vi "Constrained Non-Linear Fit (Best of All).vi"(0 "Y Array":dbl[](array[numeric]), 1 "f(x,a)":refnum<vi>, 2 "Data":variant, 3 "Fitting Method":T2=enum."Best of All", 4 "Optimal Offset Selection Criterion":T1, 5 "X Array":dbl[](array[numeric]), 7 "Weights":dbl[](array[numeric]), 9 "Guess Fitted Parameters":dbl[](array[numeric]), 11 "error in (no error)":errorcluster, 12 "Termination Criteria":T4={"Max Iterations"=1000, "Max Function Calls"=10000, "Max Time"=1000.0, "Function Tolerance"=1e-06, "Parameter Tolerance"=1e-06, "Gradient Tolerance"=1e-06, "Min Lambda"=1e-06, "Max Lambda"=1e-06, "Initial Tick Count"=0}, 13 "Fitted parameter bounds":T7, 14 "Fitting Algorithm":T3) -> (6 "Fit Output":T8={"best nonlinear fit"=[], "best fit parameters"=[], "R^2"=0.0, "RMSE"=0.0, "error out"={"status"=FALSE, "code"=0, "source"=""}, "Fitting Method"=enum."Least Square", "number of function calls"=0, "number of iterations"=0, "covariance"=[], "Chi 2"=0.0, "DOF"=0, "Fit Convergence Criterion"=enum."Continue", "Fitting Algorithm"=enum."Levenberg-Marquardt", "Weighted Fit"=enum."Unweighted", "Gradient"=0.0, "|Delta Chi 2|"=0.0, "|Delta Chi 2|/Chi 2"=0.0, "Max |Delta a| /|a|"=0.0, "Lambda"=-1.0, "RSS"=0.0, "AIC"=0.0, "BIC"=0.0, "Max number of function calls"=0, "Max number of iterations"=0, "IRF"={"X Array"=[], "Y Array"=[]}, "IRF Normalization Factor"=0.0, "Decay Normalization Factor"=0.0, "Number of offset fits"=0, "Weighted Chi2"=-1.0, "Unweighted Chi2"=-1.0}, 8 "Fit Results (Stats)":T6[](array[typedef]), 10 "Fit Aborted?":bool, 15 "Error Out":errorcluster)   [LabVIEW 2021, in "Fits.lvlib"]
uses:
  Fits.lvlib
  Non-linear Fit Output v4.ctl
  Nonlinear Fit Method.ctl
  <vilib>/Analysis/Matrix/Datatypes/RealMatrix.ctl
  Convergence Criteria.ctl
  Non-linear Fitting Algorithm.ctl
  IRF(X)PSED/Fit Weights Type v2.ctl
  Graphs/XY Graph/XY Graph Plot Data.ctl
  My Fit Stopping Criteria.ctl
  Non-linear Fitting Method v2.ctl
  Fit Results (statistics).ctl
  Optimal Offset Selection Criterion.ctl
  Decay Convolution/Fit Control Data.ctl
  Decay Convolution/Fit Control Data v2.ctl
  IRF(X)PSED/Decay Fit Parameters In List.ctl
  Decay Convolution/Decay Model.ctl
  Abort Fit Global.vi
  <userlib>/_OpenG.lib/array/array.llb/Remove Duplicates from 1D Array (DBL)__ogtk.vi
  <vilib>/Analysis/NI_AALPro.lvlib
  <vilib>/Analysis/Matrix/NI_Matrix.lvlib
  Graphs/XY Graph/XY Graph Add-Ons.lvlib
  Error/Error.lvlib
  <userlib>/_OpenG.lib/array/array.llb/openg_array.lvlib
panel:
  in  "Cluster":T5={"Optimal Offset Selection Criterion"=enum."Min Chi^2", "Fitting Method"=enum."Best of All", "Fitting Algorithm"=enum."Levenberg-Marquardt", "Termination Criteria"={"Max Iterations"=1000, "Max Function Calls"=10000, "Max Time"=1000.0, "Function Tolerance"=1e-06, "Parameter Tolerance"=1e-06, "Gradient Tolerance"=1e-06, "Min Lambda"=1e-06, "Max Lambda"=1e-06, "Initial Tick Count"=0}, "Fitted parameter bounds"={"parameter minimum"=[], "parameter maximum"=[]}}
  # "see the AlliGator License on the block diagram (Ctrl+E or Window:Show Block Diagram)"
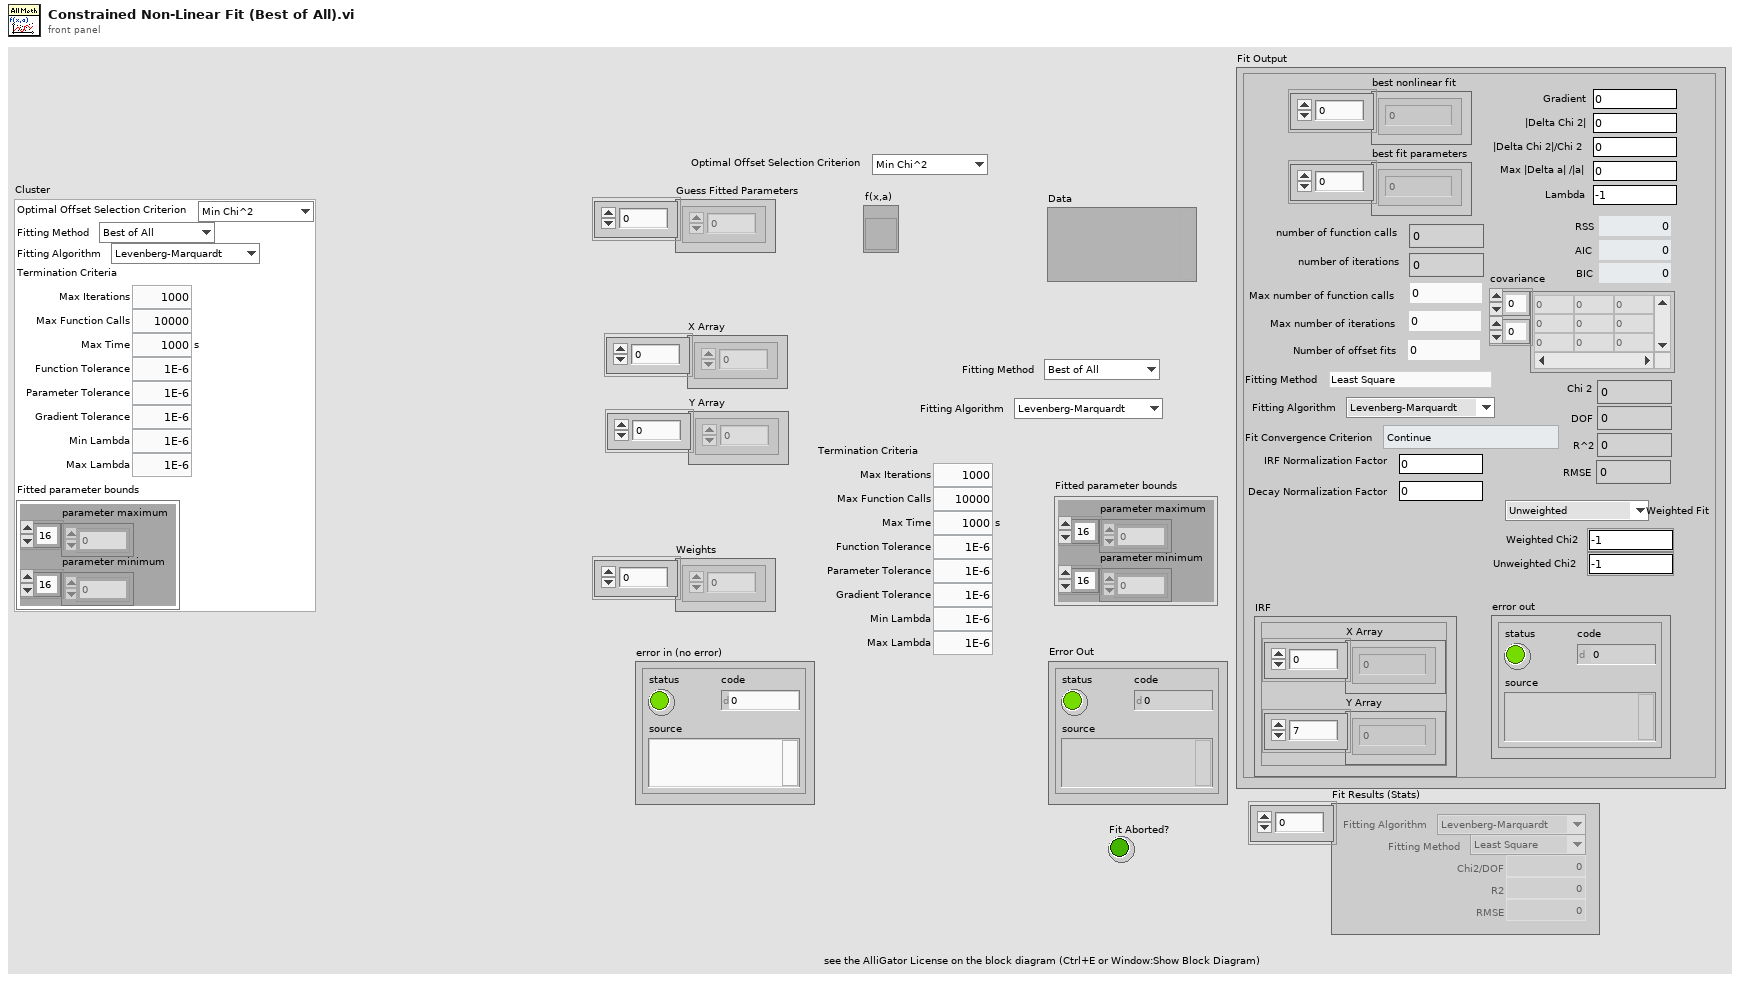
[diagram p1: front panel]
types:
  T1 = typedef "Fits.lvlib/Optimal Offset Selection Criterion.ctl" = enum16{"Min Chi^2", "Max R^2"}
  T2 = typedef "Fits.lvlib/Non-linear Fitting Method v2.ctl" = enum16{"Least Square", "Least Absolute Residual", "Bisquare", "MLE", "-", "Best of All"}
  T3 = typedef "Fits.lvlib/Non-linear Fitting Algorithm.ctl" = enum16{"Levenberg-Marquardt", "Trust-Region Dogleg"}
  T4 = typedef "Fits.lvlib/My Fit Stopping Criteria.ctl" = cluster{"Max Iterations":i32, "Max Function Calls":i32, "Max Time":dbl[unit], "Function Tolerance":dbl, "Parameter Tolerance":dbl, "Gradient Tolerance":dbl, "Min Lambda":dbl, "Max Lambda":dbl, "Initial Tick Count":u32}
  T5 = cluster{"Optimal Offset Selection Criterion":T1, "Fitting Method":T2, "Fitting Algorithm":T3, "Termination Criteria":T4, "Fitted parameter bounds":cluster{"parameter minimum":dbl[], "parameter maximum":dbl[]}}
  T6 = typedef "Fits.lvlib/Fit Results (statistics).ctl" = cluster{"Chi2/DOF":dbl, "R2":dbl, "RMSE":dbl, "Fitting Method":T2, "Fitting Algorithm":T3}
  T7 = cluster{"parameter minimum":dbl[], "parameter maximum":dbl[]}
  T8 = typedef "Fits.lvlib/Non-linear Fit Output v4.ctl" = cluster{"best nonlinear fit":dbl[], "best fit parameters":dbl[], "R^2":dbl, "RMSE":dbl, "error out":errorcluster, "Fitting Method":T9, "number of function calls":i32, "number of iterations":i32, "covariance":T10, "Chi 2":dbl, "DOF":i32, "Fit Convergence Criterion":T11, "Fitting Algorithm":T3, "Weighted Fit":T12, "Gradient":dbl, "|Delta Chi 2|":dbl, "|Delta Chi 2|/Chi 2":dbl, "Max |Delta a| /|a|":dbl, "Lambda":dbl, "RSS":dbl, "AIC":dbl, "BIC":dbl, "Max number of function calls":i32, "Max number of iterations":i32, "IRF":T13, "IRF Normalization Factor":dbl, "Decay Normalization Factor":dbl, "Number of offset fits":i32, "Weighted Chi2":dbl, "Unweighted Chi2":dbl}
  T9 = typedef "Fits.lvlib/Nonlinear Fit Method.ctl" = enum16{"Least Square", "Least Absolute Residual", "Bisquare", "MLE"}
  T10 = typedef "NI_Matrix.lvlib/RealMatrix.ctl" = dbl[][]
  T11 = typedef "Fits.lvlib/Convergence Criteria.ctl" = enum16{"Continue", "Tolerances Exceeded", "Max Time Exceeded", "Max Iterations Exceeded", "Max Function Evaluations Exceeded", "Scale Range Exceeded"}
  T12 = typedef "Fits.lvlib/Fit Weights Type v2.ctl" = enum16{"Unweighted", "1/Variance (Neyman)", "1/Variance (Pearson)", "Best of All"}
  T13 = typedef "XY Graph Add-Ons.lvlib/XY Graph Plot Data.ctl" = cluster{"X Array":dbl[], "Y Array":dbl[]}
  T14 = typedef "Fits.lvlib/Fit Control Data v2.ctl" = cluster{"IRF":T13, "Laser Period":dbl, "SYNC Period":dbl, "Fixed Parameter Names":T15[], "Fixed Parameter Values":dbl[], "Fitted Parameter Names":T15[], "Fit Model":T16}
  T15 = typedef "Fits.lvlib/Decay Fit Parameters In List.ctl" = enum16{"Offset", "Baseline", "A_1", "tau_1", "A_2", "tau_2"}
  T16 = typedef "Fits.lvlib/Decay Model.ctl" = enum16{"1-Exponential", "2-Exponentials"}
  T17 = typedef "Fits.lvlib/Fit Control Data.ctl" = cluster{"IRF":T13, "Laser Period":dbl, "SYNC Period":dbl}
  T18 = typedef "Fits.lvlib/Fit Statistics v3.ctl" = cluster{"# Iterations":i32, "# Function Calls":i32, "Chi2":dbl, "Chi2/DOF":dbl, "Fit Convergence Criterion":T11, "Gradient":dbl, "|Delta Chi 2|":dbl, "|Delta Chi 2|/Chi 2":dbl, "Max |Delta a| /|a|":dbl, "Lambda":dbl, "Weighted Chi2":dbl, "Unweighted Chi2":dbl}
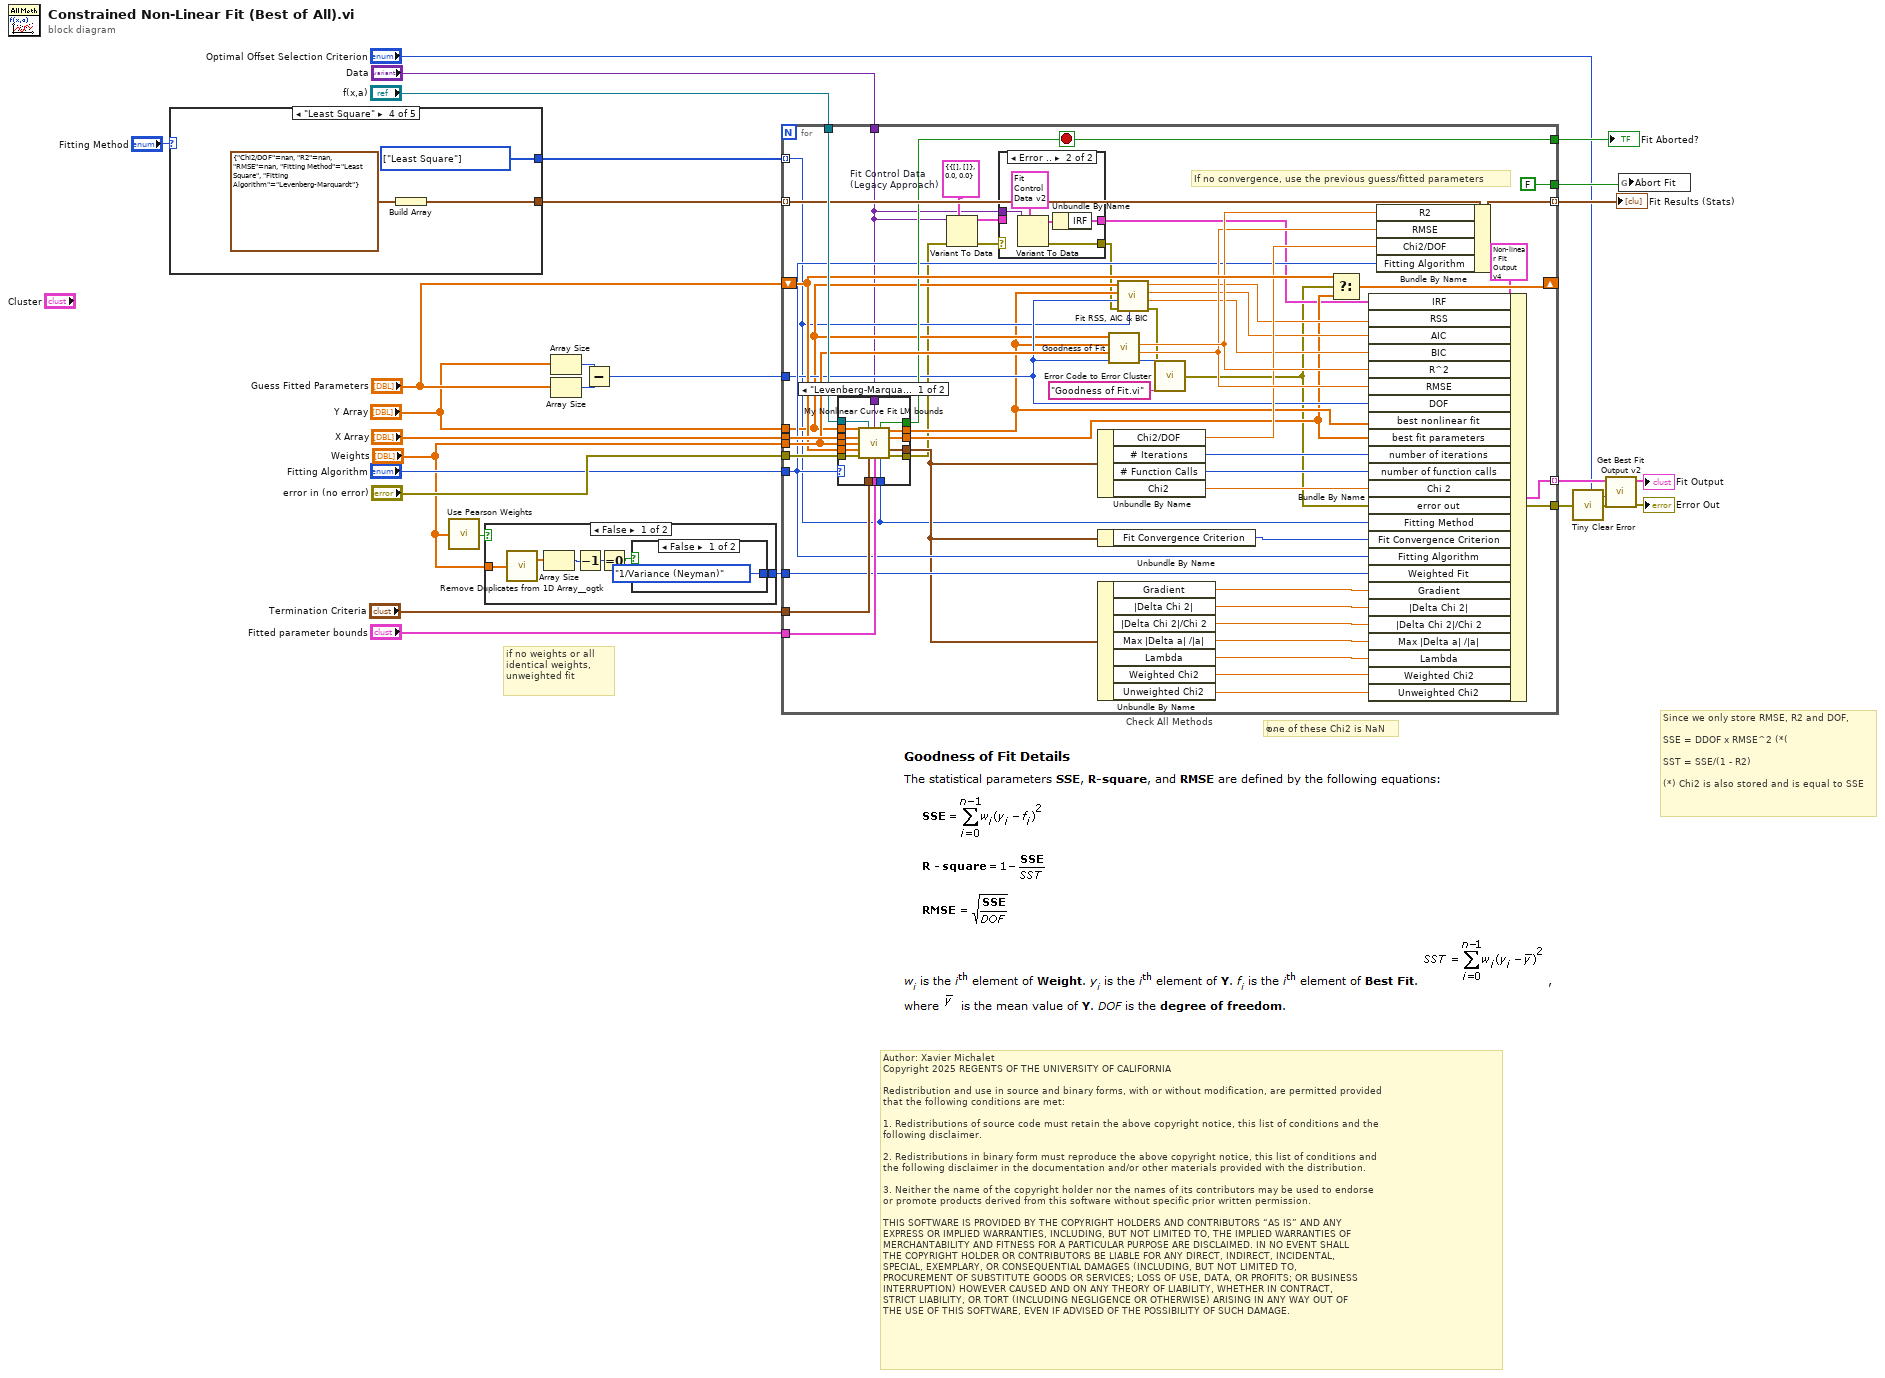
[diagram p0: block diagram]
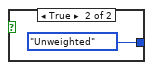
[diagram p2: hidden frame]
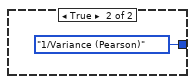
[diagram p3: hidden frame]
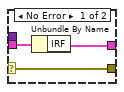
[diagram p4: hidden frame]
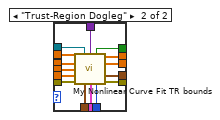
[diagram p5: hidden frame]
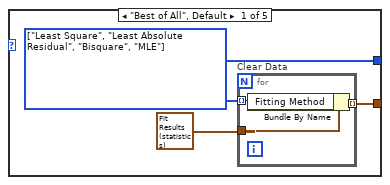
[diagram p6: hidden frame]
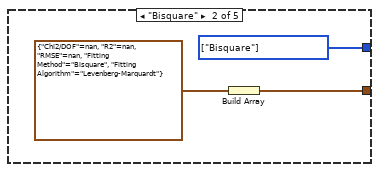
[diagram p7: hidden frame]
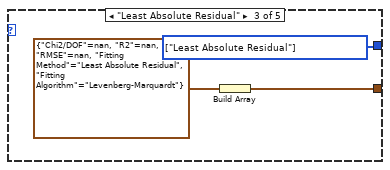
[diagram p8: hidden frame]
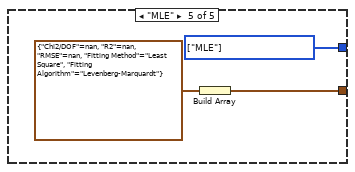
[diagram p9: hidden frame]
diagram:
  # "one of these Chi2 is NaN"
  # "one of these Chi2 is NaN"
  # "Author: Xavier Michalet\nCopyright 2025 REGENTS OF THE UNIVERSITY OF CALIFORNIA\n\nRedistribution and use in source and binary forms, with or without modification, are permitted provided\nthat the following conditions are met:\n\n1. Redistributions of source code must retain the above copyright notice, this list of conditions and the\nfollowing disclaimer.\n\n2. Redistributions in binary form must reproduce the above copyright notice, this list of conditions and\nthe following disclaimer in the documentation and/or other materials provided with the distribution.\n\n3. Neither the name of the copyright holder nor the names of its contributors may be used to endorse \nor promote products derived from this software without specific prior written permission.\n\nTHIS SOFTWARE IS PROVIDED BY THE COPYRIGHT HOLDERS AND CONTRIBUTORS “AS IS” AND ANY \nEXPRESS OR IMPLIED WARRANTIES, INCLUDING, BUT NOT LIMITED TO, THE IMPLIED WARRANTIES OF\nMERCHANTABILITY AND FITNESS FOR A PARTICULAR PURPOSE ARE DISCLAIMED. IN NO EVENT SHALL\nTHE COPYRIGHT HOLDER OR CONTRIBUTORS BE LIABLE FOR ANY DIRECT, INDIRECT, INCIDENTAL, \nSPECIAL, EXEMPLARY, OR CONSEQUENTIAL DAMAGES (INCLUDING, BUT NOT LIMITED TO, \nPROCUREMENT OF SUBSTITUTE GOODS OR SERVICES; LOSS OF USE, DATA, OR PROFITS; OR BUSINESS\nINTERRUPTION) HOWEVER CAUSED AND ON ANY THEORY OF LIABILITY, WHETHER IN CONTRACT, \nSTRICT LIABILITY, OR TORT (INCLUDING NEGLIGENCE OR OTHERWISE) ARISING IN ANY WAY OUT OF\nTHE USE OF THIS SOFTWARE, EVEN IF ADVISED OF THE POSSIBILITY OF SUCH DAMAGE."
  # "if no weights or all identical weights, unweighted fit"
  # "Since we only store RMSE, R2 and DOF,\n\nSSE = DDOF x RMSE^2 (*(\n\nSST = SSE/(1 - R2)\n\n(*) Chi2 is also stored and is equal to SSE"
  n1 = case shown="\"Least Square\"" "Fitting Method" {
    tunnel: [w30 w36 w39 w42 w45] -> w11
    tunnel: [w29 w35 w38 w41 w44] -> w9
    frame "Best of All", Default {
      w30 = T9[] [enum."Least Square", enum."Least Absolute Residual", enum."Bisquare", enum."MLE"] items=["Least Square", "Least Absolute Residual", "Bisquare", "MLE"] ("Array")
      n2 = for "Clear Data" {
        tunnel: w30 -> [w32] mode=indexing
        tunnel: T6 {"Chi2/DOF"=nan, "R2"=nan, "RMSE"=nan, "Fitting Method"=enum."Least Square", "Fitting Algorithm"=enum."Levenberg-Marquardt"} ("Fit Statistics") -> [w33]
        tunnel: [w31] -> w29 mode=indexing
        n3 = Bundle By Name(cluster=w33, "Fitting Method"=w32) -> (w31:T6)
      }
    }
    frame "Bisquare" {
      w36 = T9[] [enum."Bisquare"] items=["Least Square", "Least Absolute Residual", "Bisquare", "MLE"] ("Array")
      n4 = Build Array(T6 {"Chi2/DOF"=nan, "R2"=nan, "RMSE"=nan, "Fitting Method"=enum."Bisquare", "Fitting Algorithm"=enum."Levenberg-Marquardt"} ("Fit Statistics")) -> (w35:T6[])
    }
    frame "Least Absolute Residual" {
      w39 = T9[] [enum."Least Absolute Residual"] items=["Least Square", "Least Absolute Residual", "Bisquare", "MLE"] ("Array")
      n5 = Build Array(T6 {"Chi2/DOF"=nan, "R2"=nan, "RMSE"=nan, "Fitting Method"=enum."Least Absolute Residual", "Fitting Algorithm"=enum."Levenberg-Marquardt"} ("Fit Statistics")) -> (w38:T6[])
    }
    frame "Least Square" {
      w42 = T9[] [enum."Least Square"] items=["Least Square", "Least Absolute Residual", "Bisquare", "MLE"] ("Array")
      n6 = Build Array(T6 {"Chi2/DOF"=nan, "R2"=nan, "RMSE"=nan, "Fitting Method"=enum."Least Square", "Fitting Algorithm"=enum."Levenberg-Marquardt"} ("Fit Statistics")) -> (w41:T6[])
    }
    frame "MLE" {
      w45 = T9[] [enum."MLE"] items=["Least Square", "Least Absolute Residual", "Bisquare", "MLE"] ("Array")
      n7 = Build Array(T6 {"Chi2/DOF"=nan, "R2"=nan, "RMSE"=nan, "Fitting Method"=enum."Least Square", "Fitting Algorithm"=enum."Levenberg-Marquardt"} ("Fit Statistics")) -> (w44:T6[])
    }
  }
  n8 = call "Use Pearson Weights.vi"("Weight"="Weights") -> ("Use Pearson Weight"=w1:bool)
  n9 = case shown="False" w1 {
    tunnel: [w47 Fit_Weights_Type_v2."1/Variance (Pearson)" ("Weighted Fit")] -> w3
    tunnel: "Weights" -> [w46 _]
    frame False {
      n10 = call-poly <userlib>:"Remove Duplicates from 1D Array__ogtk.vi"("Input Array"=w46) -> ("Output Array"=w51:dbl[])  [unwired: 1 out]
      n11 = Array Size(array=w51) -> (size(s)=w50:i32)
      n12 = Decrement(x=w50) -> (x-1=w49:i32)
      n13 = Equal To 0?(x=w49) -> (x = 0?=w48:bool)
      n14 = case shown="False" w48 {
        tunnel: [Fit_Weights_Type_v2."1/Variance (Neyman)" ("Weighted Fit") Fit_Weights_Type_v2."Unweighted" ("Weighted Fit")] -> w47
        frame False {
        }
        frame True {
        }
      }
    }
    frame True {
    }
  }
  n15 = Array Size(array="Y Array") -> (size(s)=w17:i32)
  n16 = Array Size(array="Guess Fitted Parameters") -> (size(s)=w18:i32)
  n17 = Subtract(x=w17, y=w18) -> (x-y=w24:i32)
  n18 = for "Check All Methods" {
    tunnel: "Y Array" -> [w74]
    tunnel: "X Array" -> [w104]
    tunnel: "Weights" -> [w101]
    shift-right: [w98] -> _
    shift-left: "Guess Fitted Parameters" -> [w99]
    tunnel: "f(x,a)" -> [w102]
    tunnel: "Data" -> [w58]
    tunnel: w11 -> [w70] mode=indexing
    tunnel: w24 -> [w75]
    tunnel: [w100] -> w26 mode=indexing
    tunnel: "error in (no error)" -> [w103]
    tunnel: "Termination Criteria" -> [w89]
    tunnel: "Fitted parameter bounds" -> [w97]
    tunnel: [w84] -> w13
    tunnel: [FALSE ("Abort Fit")] -> w10
    tunnel: w9 -> [w88] mode=indexing
    tunnel: [w87] -> w8 mode=indexing
    tunnel: "Fitting Algorithm" -> [w83]
    tunnel: w3 -> [w82]
    tunnel: [w63] -> w6
    stop <- w84 stop-if-true
    w61 = T17 {"IRF"={"X Array"=[], "Y Array"=[]}, "Laser Period"=0.0, "SYNC Period"=0.0}  # Fit Control Data (Legacy Approach)
    # "If no convergence, use the previous guess/fitted parameters"
    n19 = case shown="\"Levenberg-Marquardt\", Default" w83 {
      tunnel: w104 -> [w127 w142]
      tunnel: w103 -> [w126 w141]
      tunnel: w102 -> [w125 w140]
      tunnel: w58 -> [w124 w139]
      tunnel: w74 -> [w123 w138]
      tunnel: w101 -> [w122 w137]
      tunnel: w99 -> [w121 w136]
      tunnel: w97 -> [w120 w135]
      tunnel: [w119 w134] -> w69
      tunnel: [w118 w133] -> w68
      tunnel: [w117 w132] -> w62
      tunnel: w70 -> [w116 w131]
      tunnel: w89 -> [w115 w130]
      tunnel: [w114 w129] -> w81
      tunnel: [w113 w128] -> w84
      frame "Levenberg-Marquardt", Default {
        n20 = call "My Nonlinear Curve Fit LM bounds.vi"("Y"=w123, "f(x,a)"=w125, "data"=w124, "X"=w127, "Weight"=w122, "initial parameters"=w121, "error in (no error)"=w126, "Termination Criteria"=w115, "parameter bounds"=w120, "NL Fit Method"=w116) -> ("Fit Aborted?"=w113:bool, "best nonlinear fit"=w119:dbl[], "best fit parameters"=w118:dbl[], "Fit Statistics"=w114:T18, "error out"=w117:errorcluster)  [unwired: 1 out]
      }
      frame "Trust-Region Dogleg" {
        n21 = call "My Nonlinear Curve Fit TR bounds.vi"("Y"=w138, "f(x,a)"=w140, "data"=w139, "X"=w142, "Weight"=w137, "initial parameters"=w136, "error in (no error)"=w141, "Termination Criteria"=w130, "parameter bounds"=w135, "method"=w131) -> ("Fit Aborted?"=w128:bool, "best nonlinear fit"=w134:dbl[], "best fit parameters"=w133:dbl[], "Fit Statistics"=w129:T18, "error out"=w132:errorcluster)  [unwired: 1 out]
      }
    }
    n22 = Variant To Data(error in=w62, type=w61, Variant=w58) -> (data=w59:T17, error out=w60:errorcluster)
    n23 = case shown="Error .." w60 {
      selector: w60 -> [w105 _]
      tunnel: [w106 w110] -> w67
      tunnel: [w105 w109] -> w66
      tunnel: w59 -> [w107 _]
      tunnel: w58 -> [_ w108]
      frame No Error {
        n24 = Unbundle By Name(w107) -> ("IRF"=w106:T13)
      }
      frame Error {
        n25 = Variant To Data(type=T14 {"IRF"={"X Array"=[], "Y Array"=[]}, "Laser Period"=0.0, "SYNC Period"=0.0, "Fixed Parameter Names"=[], "Fixed Parameter Values"=[], "Fitted Parameter Names"=[], "Fit Model"=enum."1-Exponential"} ("Fit Control Data"), Variant=w108) -> (data=w111:T14, error out=w109:errorcluster)  [unwired: 1 in]
        n26 = Unbundle By Name(w111) -> ("IRF"=w110:T13)
      }
    }
    n27 = Unbundle By Name(w81) -> ("Chi2/DOF"=w93:dbl, "# Iterations"=w92:i32, "# Function Calls"=w91:i32, "Chi2"=w86:dbl)
    n28 = Unbundle By Name(w81) -> ("Fit Convergence Criterion"=w85:T11)
    n29 = Unbundle By Name(w81) -> ("Gradient"=w80:dbl, "|Delta Chi 2|"=w79:dbl, "|Delta Chi 2|/Chi 2"=w78:dbl, "Max |Delta a| /|a|"=w77:dbl, "Lambda"=w76:dbl, "Weighted Chi2"=w56:dbl, "Unweighted Chi2"=w55:dbl)
    n30 = call <vilib>:"Goodness of Fit.vi"("degree of freedom"=w75, "Weight"=w101, "Best Fit"=w69, "Y"=w74) -> ("error"=w65:i32, "RMSE"=w94:dbl, "R-square"=w95:dbl)  [unwired: 4 in, 1 out]
    n31 = call "Fit RSS, AIC & BIC.vi"("NL Fit Method"=w70, "Error In"=w66, "DOF"=w75, "Best Fit"=w69, "Data"=w74) -> ("Error Out"=w64:errorcluster, "BIC"=w71:dbl, "AIC"=w72:dbl, "RSS"=w73:dbl)  [unwired: 3 in]
    n32 = call "Error Code to Error Cluster.vi"("Error Code"=w65, "Error Source"="Goodness of Fit.vi", "Error In"=w64) -> ("Error Out"=w63:errorcluster)  [unwired: 12 in]
    n33 = Select(t=w99, s=w63, f=w68) -> (s? t:f=w98:dbl[])
    n34 = Bundle By Name(cluster=T8 {"best nonlinear fit"=[], "best fit parameters"=[], "R^2"=0.0, "RMSE"=0.0, "error out"={"status"=FALSE, "code"=0, "source"=""}, "Fitting Method"=enum."Least Square", "number of function calls"=0, "number of iterations"=0, "covariance"=[], "Chi 2"=0.0, "DOF"=0, "Fit Convergence Criterion"=enum."Continue", "Fitting Algorithm"=enum."Levenberg-Marquardt", "Weighted Fit"=enum."Unweighted", "Gradient"=0.0, "|Delta Chi 2|"=0.0, "|Delta Chi 2|/Chi 2"=0.0, "Max |Delta a| /|a|"=0.0, "Lambda"=-1.0, "RSS"=0.0, "AIC"=0.0, "BIC"=0.0, "Max number of function calls"=0, "Max number of iterations"=0, "IRF"={"X Array"=[], "Y Array"=[]}, "IRF Normalization Factor"=0.0, "Decay Normalization Factor"=0.0, "Number of offset fits"=0, "Weighted Chi2"=-1.0, "Unweighted Chi2"=-1.0} ("NL Fit Output"), "IRF"=w67, "RSS"=w73, "AIC"=w72, "BIC"=w71, "R^2"=w95, "RMSE"=w94, "DOF"=w75, "best nonlinear fit"=w69, "best fit parameters"=w68, "number of iterations"=w92, "number of function calls"=w91, "Chi 2"=w86, "error out"=w63, "Fitting Method"=w70, "Fit Convergence Criterion"=w85, "Fitting Algorithm"=w83, "Weighted Fit"=w82, "Gradient"=w80, "|Delta Chi 2|"=w79, "|Delta Chi 2|/Chi 2"=w78, "Max |Delta a| /|a|"=w77, "Lambda"=w76, "Weighted Chi2"=w56, "Unweighted Chi2"=w55) -> (w100:T8)
    n35 = Bundle By Name(cluster=w88, "R2"=w95, "RMSE"=w94, "Chi2/DOF"=w93, "Fitting Algorithm"=w83) -> (w87:T6)
  }
  "Fit Aborted?" <- w13
  "Fit Results (Stats)" <- w8
  n36 = call "Tiny Clear Error.vi"("Error In"=w6) -> ("no Error Out"=w5:errorcluster)  [unwired: 8 in]
  n37 = call "Get Best Fit Output v2.vi"("error in"=w5, "Optimal Offset Selection Criterion"="Optimal Offset Selection Criterion", "Array of Fit Outputs"=w26) -> ("Error Out"=→"Error Out":errorcluster, "Best Fit Output"=→"Fit Output":T8)  [unwired: 6 in, 1 out]
  n38 = global write "Abort Fit Global.vi" "Abort Fit"(w10) -> ()
